vi "Replace Specified Characters From Multibyte Array.vi"(8 "error in (no error)":errorcluster, 9 "Replacement":string="-", 10 "Problem Characters":string[](array[string]), 11 "Array of Multibyte Characters":string[](array[string])) -> (0 "error out":errorcluster, 2 "Any Characters Removed?":bool, 3 "Modified Array":string[](array[string]))   [LabVIEW 2020, in "NI_Multibyte Utilities.lvlib"]
doc: "Replace any of the problem multibyte characters found in the multibyte character array with the replacement character (default is hyphen)."
uses:
  <vilib>/Utility/Multibyte/NI_Multibyte Utilities.lvlib
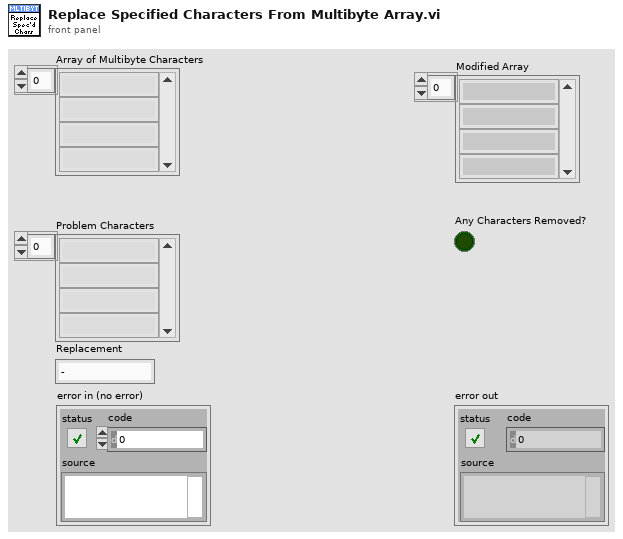
[diagram p1: front panel]
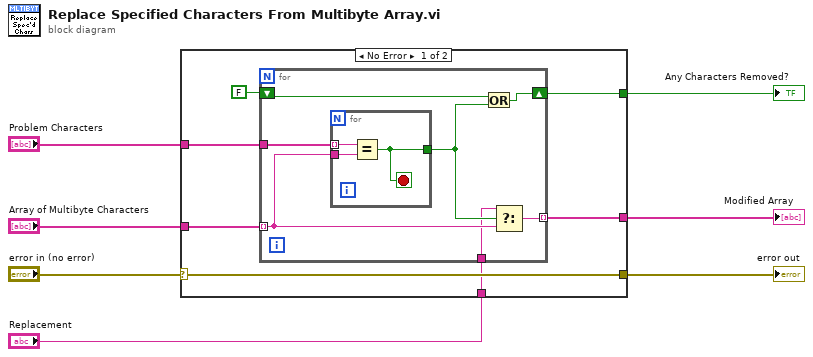
[diagram p0: block diagram]
diagram:
  n1 = case shown="No Error" "error in (no error)" {
    selector: "error in (no error)" -> [w12 w25]
    tunnel: "Array of Multibyte Characters" -> [w10 _]
    tunnel: [w12 w25] -> w7
    tunnel: "Problem Characters" -> [w11 _]
    tunnel: [w13 _] -> w5
    tunnel: [w9 _] -> w4
    tunnel: "Replacement" -> [w8 _]
    frame No Error {
      n2 = for {
        tunnel: w10 -> [w17] mode=indexing
        tunnel: w11 -> [w21]
        shift-right: [w19] -> w13
        shift-left: FALSE -> [w20]
        tunnel: [w16] -> w9 mode=indexing
        tunnel: w8 -> [w15]
        n3 = for {
          tunnel: w21 -> [w24] mode=indexing
          tunnel: w17 -> [w23]
          tunnel: [w22] -> w18
          stop <- w22 stop-if-true
          n4 = Equal?(x=w24, y=w23) -> (x = y?=w22:bool)
        }
        n5 = Or(x=w20, y=w18) -> (x .or. y?=w19:bool)
        n6 = Select(t=w15, s=w18, f=w17) -> (s? t:f=w16:string)
      }
    }
    frame Error {
    }
  }
  "error out" <- w7
  "Any Characters Removed?" <- w5
  "Modified Array" <- w4
